vi "RH Probe Global Var.vi"() -> ()   [LabVIEW 2011]
panel:
  out "# RH Probes Indicator":dbl
  in  "# RH Probes":dbl
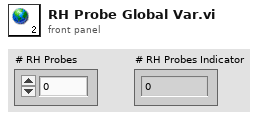
[diagram p1: front panel]
diagram:
